vi "Initiate.vi"   [LabVIEW 2018, in "Agilent U2000 Series.lvlib"]
doc: "Initiates a measurement based on the preset configuration. The measurement type must be configured before calling this function. This is accomplished by calling the Configure Measurement VI. After the Initiate VI is called, the Power Meter leaves the Idle state and waits for a trigger.\n\nNote:\nUse this VI only with other low-level VIs. The high-level VIs automatically incorporate this functionality. This VI does not check the instrument status."
uses:
  Agilent U2000 Series.lvlib
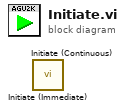
[diagram p0: block diagram]
diagram:
  n1 = call "Initiate (Immediate).vi"() -> ()  [unwired: 10 in, 2 out]
  n2 = call "Initiate (Continuous).vi"() -> ()  [unwired: 10 in, 2 out]
